vi "TMYTEK_FPGA_Ctrl.vi"() -> ()   [LabVIEW 2019]
uses:
  <vilib>/Platform/TimedLoop/XDataNode/timing_clust.ctl
  <vilib>/Platform/TimedLoop/XDataNode/nitl_modes.ctl
  <vilib>/Platform/TimedLoop/XDataNode/wakeup.ctl
  <vilib>/rvi/Emulation/niFpgaGetClockAttributes.vi
  <vilib>/rvi/Emulation/niFpgaSctlEmulationGetInTimedLoop.vi
  <vilib>/rvi/Emulation/niFpgaEmulationReportErrorSimple.vi
  <vilib>/rvi/eio/common/nirviEmuTemplateMethod_errors.vi
  <vilib>/rvi/Emulation/niFpgaCriticalErrorInLSC.vi
  <vilib>/rvi/interface/RandomDataEmulation/niFpgaRandomDataHandleErrors.vi
  <vilib>/eio/EIONode/EIONode.xnode
  <vilib>/platform/TimedLoop/XDataNode/XDataNode.xnode
  <vilib>/rvi/DataTransferAndStorage/Container/XNode/niFpgaContainer.xnode
  <vilib>/rvi/interface/RandomDataEmulation/nirviRandomDataFpgaReadWriteTemplate.vi
  <vilib>/Platform/TimedLoop/XDataNode/XDNodeRunTimeDep.lvlib
panel:
  in  "AUX I/O 7":bool
  in  "AUX I/O 6":bool
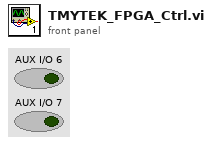
[diagram p1: front panel]
types:
  T1 = typedef "XDNodeRunTimeDep.lvlib/timing_clust.ctl" = cluster{"Expected End [f-1]":u64, "Actual End [f-1]":u64, "Finished Late? [f-1]":bool, "Expected End [i-1]":u64, "Actual End [i-1]":u64, "Finished Late? [i-1]":bool, "Expected Start [i]":u64, "Actual Start [i]":u64, "Expected Start [f]":u64, "Actual Start [f]":u64, "Source Name":string, "Structure Name":string, "Period":i64, "Deadline":i64, "Offset":i64, "Start":i64, "Priority":i32, "Timeout":i32, "Mode":T2, "Wakeup Reason":T3, "Error":errorcluster, "Source Type":string, "Secondary Source Type":string, "Global End Time":u64, "Global Start Time":u64, "Frame Duration":u64, "Iteration Duration":u64, "Assigned CPU":i32, "I/O Scan Engine Mode":u32}
  T2 = typedef "XDNodeRunTimeDep.lvlib/nitl_modes.ctl" = enum32{"No Change", "Process missed periods, maintain original phase", "Discard missed periods, maintain original phase", "Process missed periods, ignore original phase", "Discard missed periods, ignore original phase"}
  T3 = typedef "XDNodeRunTimeDep.lvlib/wakeup.ctl" = enum32{"Normal", "Aborted", "Asynchronous wakeup", "Timing source error", "Timed loop error", "Timeout"}
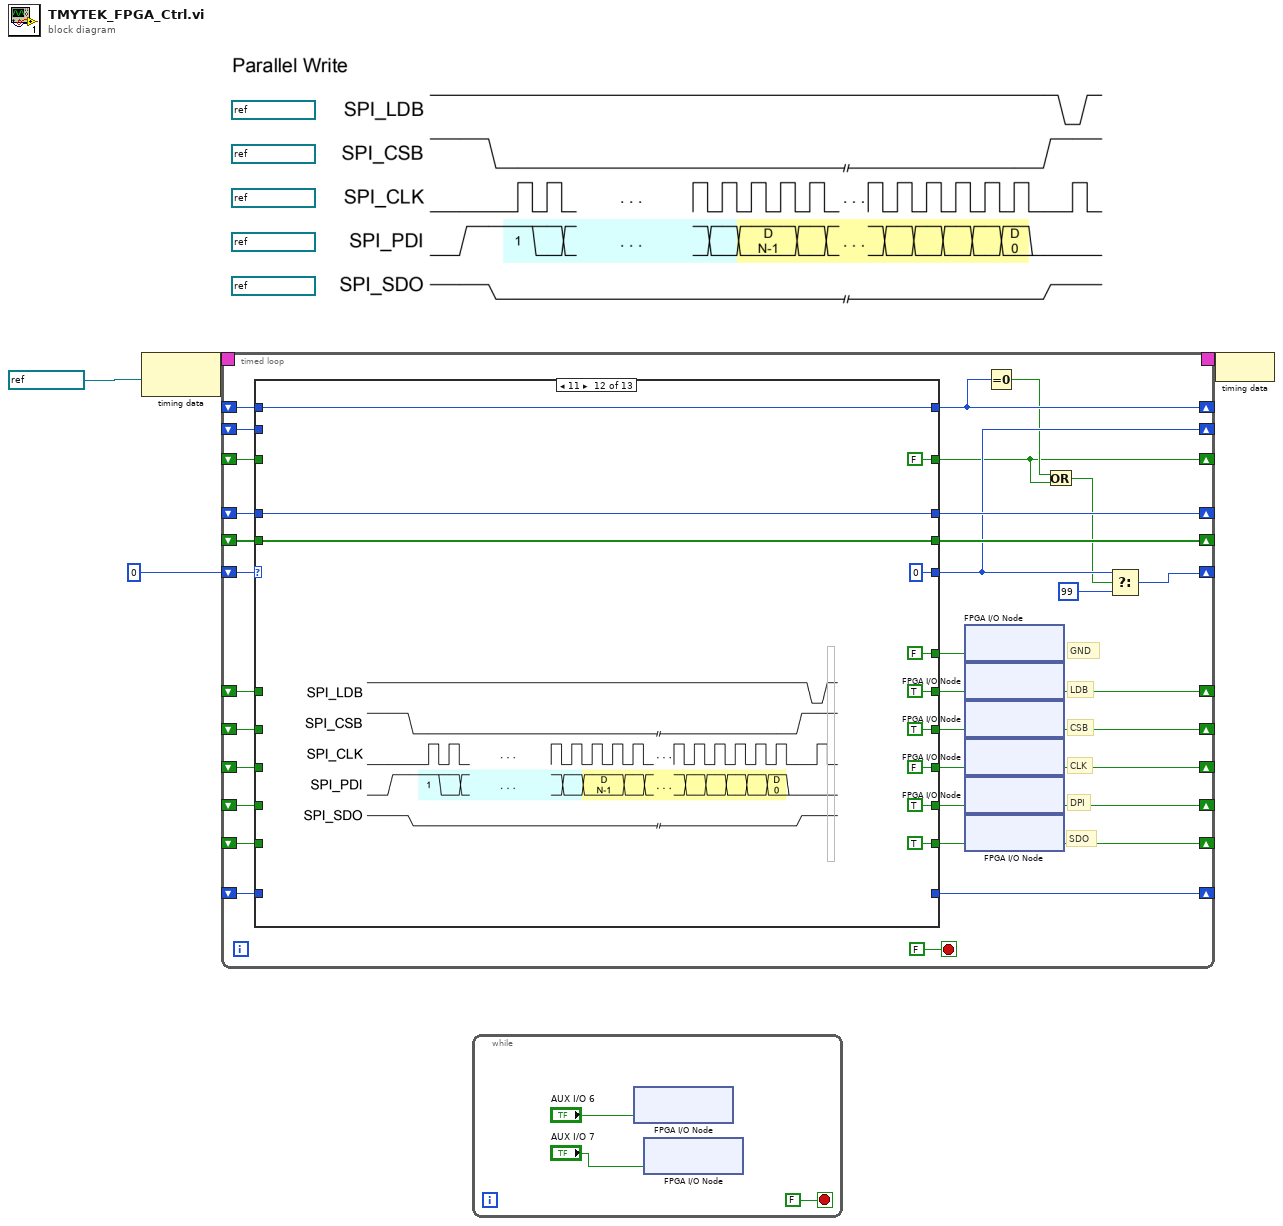
[diagram p0: block diagram]
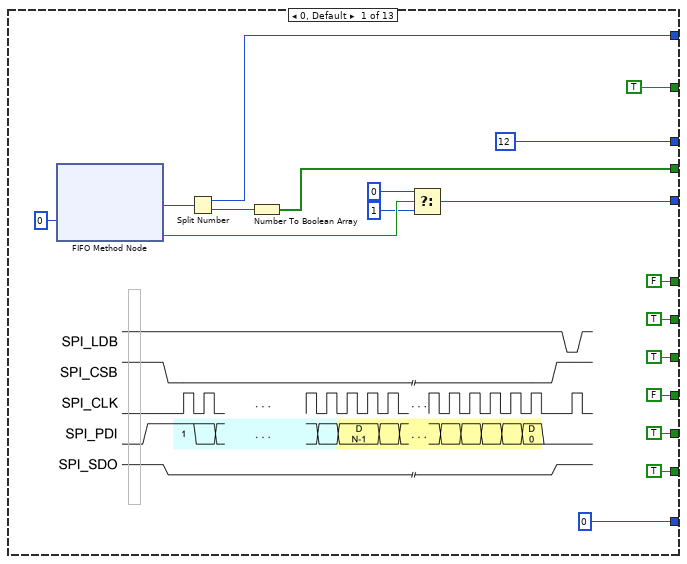
[diagram p2: hidden frame]
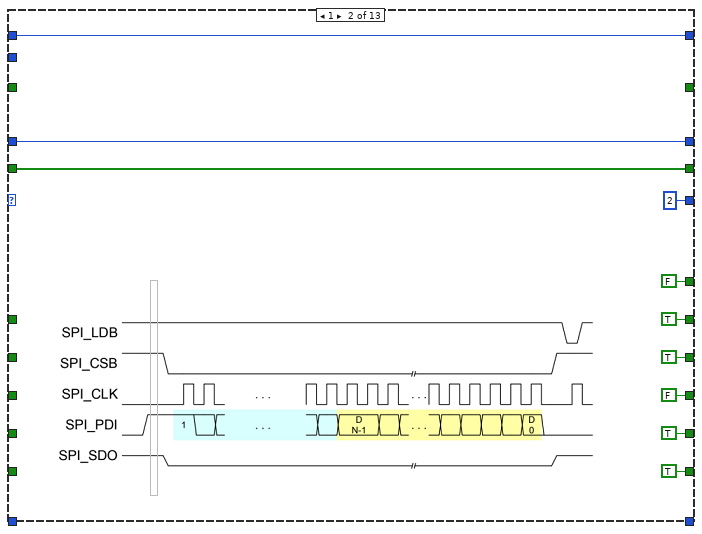
[diagram p3: hidden frame]
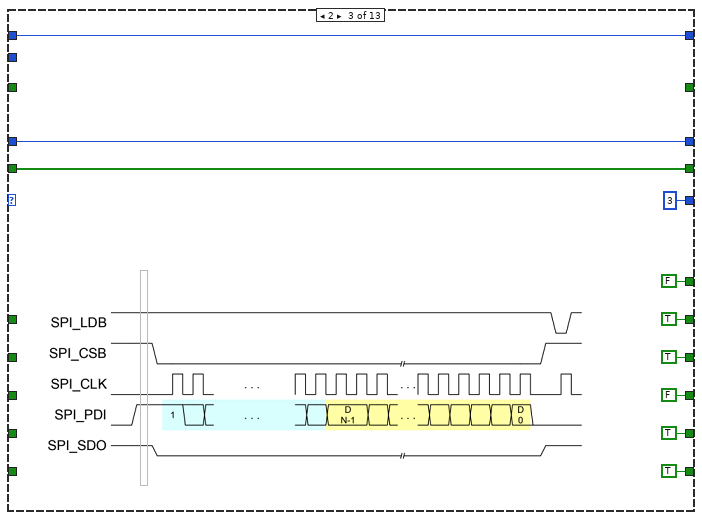
[diagram p4: hidden frame]
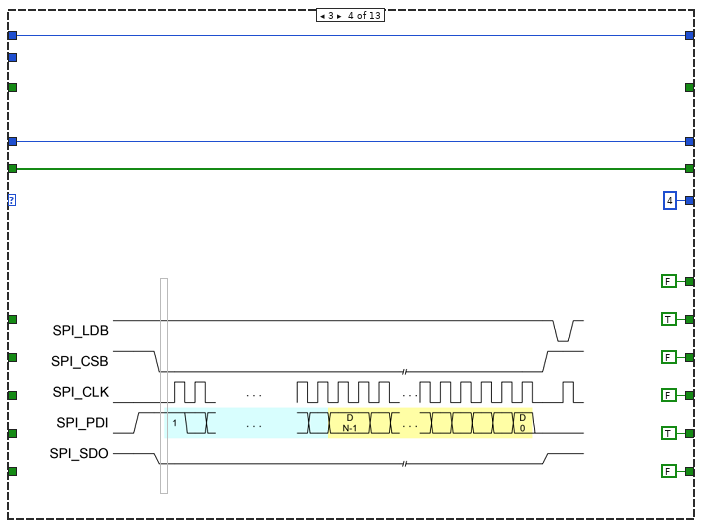
[diagram p5: hidden frame]
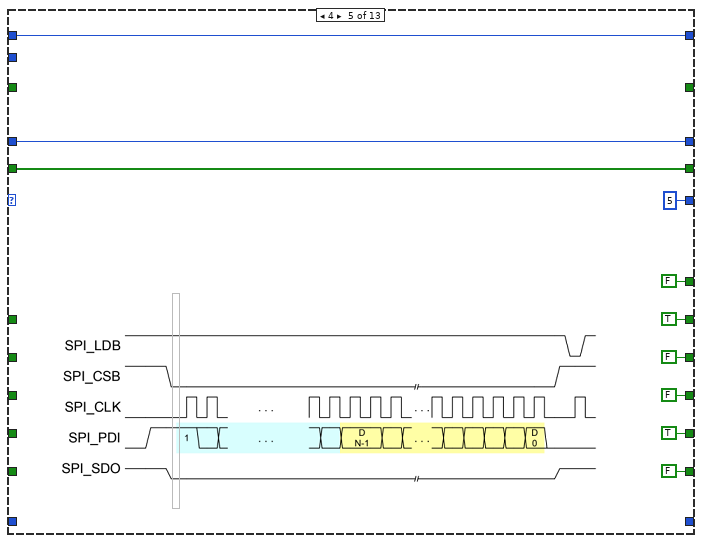
[diagram p6: hidden frame]
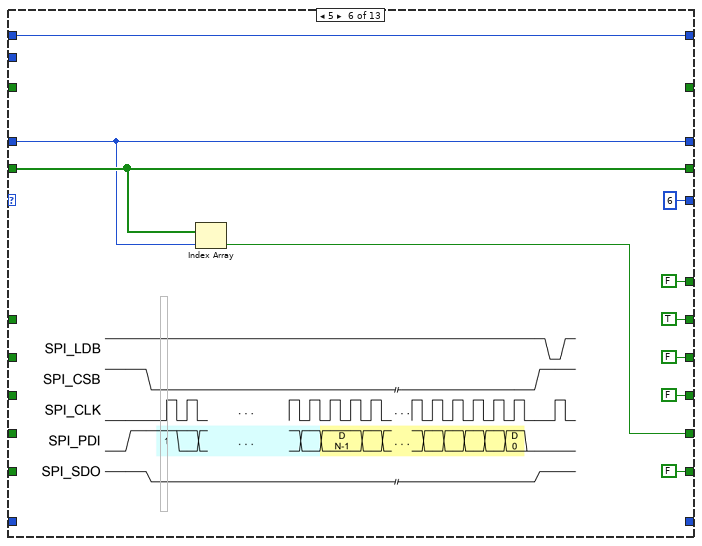
[diagram p7: hidden frame]
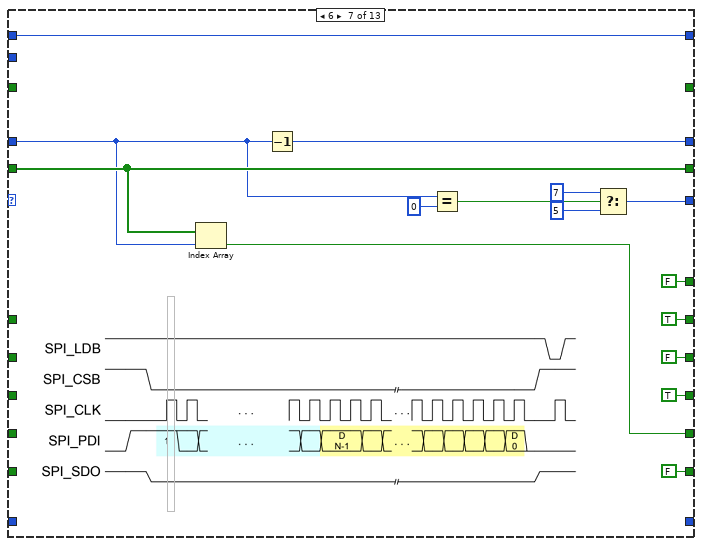
[diagram p8: hidden frame]
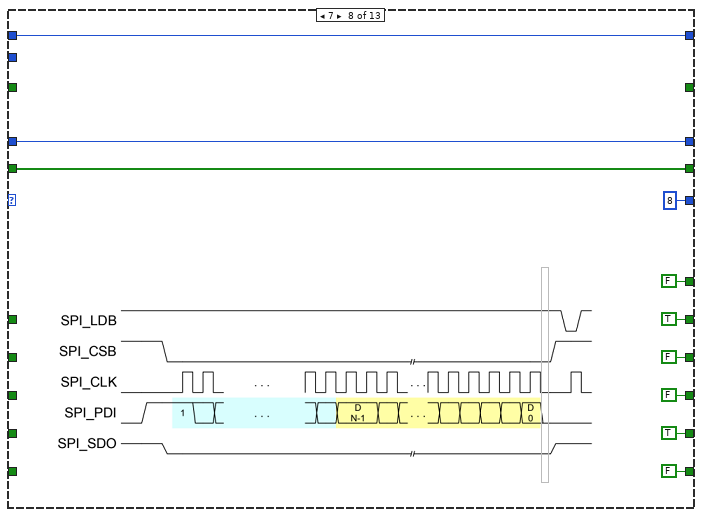
[diagram p9: hidden frame]
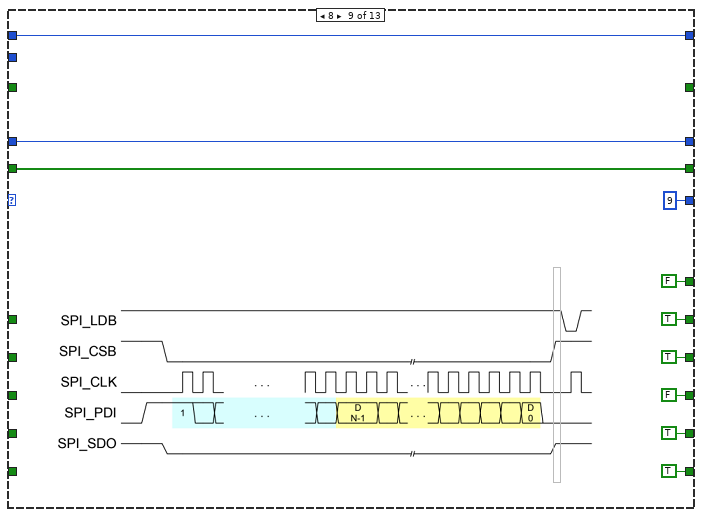
[diagram p10: hidden frame]
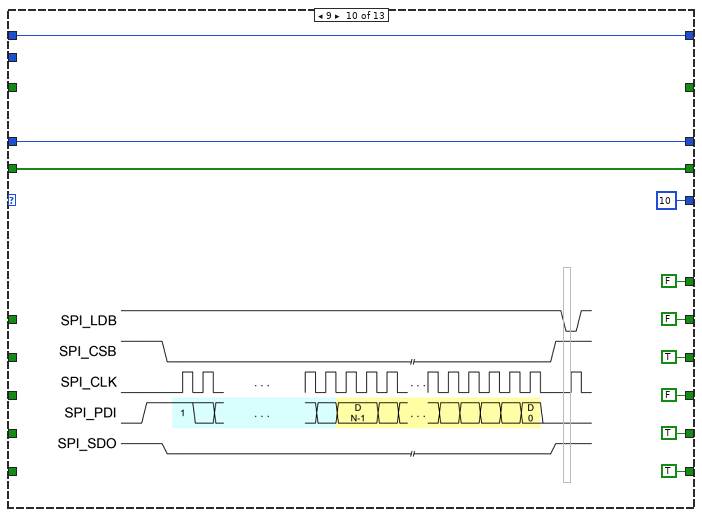
[diagram p11: hidden frame]
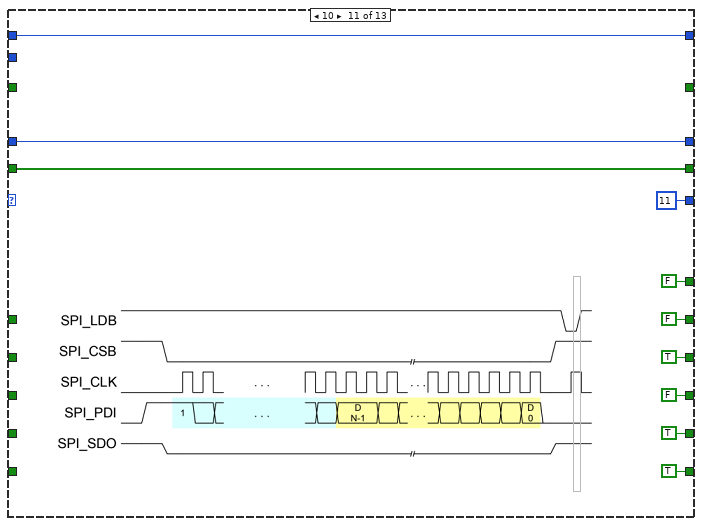
[diagram p12: hidden frame]
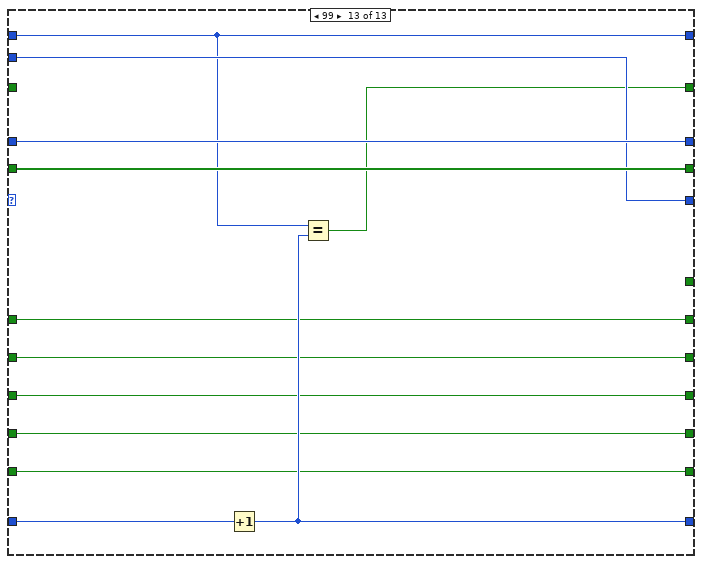
[diagram p13: hidden frame]
diagram:
  (unwired) refnum<k21> "AUX I/O 5" ("FPGA I/O")
  (unwired) refnum<k21> "AUX I/O 4" ("FPGA I/O")
  (unwired) refnum<k21> "AUX I/O 3" ("FPGA I/O")
  (unwired) refnum<k21> "AUX I/O 2" ("FPGA I/O")
  (unwired) refnum<k21> "AUX I/O 1" ("FPGA I/O")
  n1 = node-c288(refnum<k21> "120MHz" ("Source Name")) -> (w4:T1)
  n2 = timed-loop {
    timing: w4 -> [_]
    timing-out: [_] -> w3
    shift-right: [w24] -> _
    shift-left: i16 0 -> [w32]
    shift-right: [w31] -> _
    shift-left: _ -> [w30]
    shift-right: [w28] -> _
    shift-left: _ -> [w27]
    shift-right: [w23] -> _
    shift-left: _ -> [w22]
    shift-right: [w6] -> _
    shift-left: _ -> [w26]
    shift-right: [w21] -> _
    shift-left: _ -> [w20]
    shift-right: [w15] -> _
    shift-left: _ -> [w14]
    shift-right: [w16] -> _
    shift-left: _ -> [w13]
    shift-right: [w17] -> _
    shift-left: _ -> [w12]
    shift-right: [w18] -> _
    shift-left: _ -> [w11]
    shift-right: [w19] -> _
    shift-left: _ -> [w10]
    shift-right: [w8] -> _
    shift-left: _ -> [w9]
    stop <- FALSE stop-if-true
    # "SDO"
    # "DPI"
    # "CLK"
    # "GND"
    # "CSB"
    # "LDB"
    n3 = case shown="11" w32 {
      tunnel: [w47 i16 2 i16 3 i16 4 i16 5 i16 6 w103 i16 8 i16 9 i16 10 i16 11 i16 0 w177] -> w23
      tunnel: [w46 w61 w71 w81 w91 w99 w115 w119 w129 w139 w149 w160 w178] -> w31
      tunnel: w30 -> [_ w61 w71 w81 w91 w99 w115 w119 w129 w139 w149 w160 w178]
      tunnel: [FALSE FALSE FALSE FALSE FALSE FALSE FALSE FALSE FALSE FALSE FALSE FALSE _] -> w29
      tunnel: [TRUE TRUE TRUE TRUE TRUE TRUE TRUE TRUE TRUE FALSE FALSE TRUE w173] -> w15
      tunnel: [TRUE TRUE TRUE FALSE FALSE FALSE FALSE FALSE TRUE TRUE TRUE TRUE w172] -> w16
      tunnel: [FALSE FALSE FALSE FALSE FALSE FALSE TRUE FALSE FALSE FALSE FALSE FALSE w171] -> w17
      tunnel: [TRUE TRUE TRUE TRUE TRUE w97 w114 TRUE TRUE TRUE TRUE TRUE w170] -> w18
      tunnel: [TRUE TRUE TRUE FALSE FALSE FALSE FALSE FALSE TRUE TRUE TRUE TRUE w169] -> w19
      tunnel: [12 w55 w65 w77 w87 w98 w109 w126 w136 w146 w156 w167 w179] -> w28
      tunnel: w27 -> [_ w55 w65 w77 w87 w98 w108 w126 w136 w146 w156 w167 w179]
      tunnel: w26 -> [_ _ _ _ _ _ _ _ _ _ _ _ _]
      tunnel: [TRUE _ _ _ _ _ _ _ _ _ _ FALSE w174] -> w6
      tunnel: w22 -> [_ _ _ _ _ _ _ _ _ _ _ _ w177]
      tunnel: [u16 0 _ _ _ _ _ _ _ _ _ _ _ w175] -> w21
      tunnel: w20 -> [_ _ _ _ _ _ _ _ _ _ _ _ w176]
      tunnel: w14 -> [_ _ _ _ _ _ _ _ _ _ _ _ w173]
      tunnel: w13 -> [_ _ _ _ _ _ _ _ _ _ _ _ w172]
      tunnel: w12 -> [_ _ _ _ _ _ _ _ _ _ _ _ w171]
      tunnel: w11 -> [_ _ _ _ _ _ _ _ _ _ _ _ w170]
      tunnel: w10 -> [_ _ _ _ _ _ _ _ _ _ _ _ w169]
      tunnel: [w34 w52 w62 w72 w82 w92 w102 w117 w127 w137 w147 w158 w168] -> w8
      tunnel: w9 -> [_ w52 w62 w72 w82 w92 w102 w117 w127 w137 w147 w158 w168]
      frame 0, Default {
        n4 = xnode ("FIFO Method Node")("Timeout"=0) -> ("Element"=w36:u32, "Timed Out?"=w50:bool)  [unwired: 1 in, 1 out]
        n5 = Split Number(x=w36) -> (hi(x)=w34:u16, lo(x)=w35:u16)
        n6 = Number To Boolean Array(number=w35) -> (Boolean array=w46:bool[])
        n7 = Select(t=i16 0, s=w50, f=i16 1) -> (s? t:f=w47:i16)
      }
      frame 1 {
      }
      frame 2 {
      }
      frame 3 {
      }
      frame 4 {
      }
      frame 5 {
        n8 = Index Array(array=w99, index=w98) -> (element=w97:bool)
      }
      frame 6 {
        n9 = Index Array(array=w115, index=w108) -> (element=w114:bool)
        n10 = Decrement(x=w108) -> (x-1=w109:i32)
        n11 = Equal?(x=w108, y=0) -> (x = y?=w106:bool)
        n12 = Select(t=i16 7, s=w106, f=i16 5) -> (s? t:f=w103:i16)
      }
      frame 7 {
      }
      frame 8 {
      }
      frame 9 {
      }
      frame 10 {
      }
      frame 11 {
      }
      frame 99 {
        n13 = Increment(x=w176) -> (x+1=w175:u16)
        n14 = Equal?(x=w168, y=w175) -> (x = y?=w174:bool)
      }
    }
    n15 = xnode "FPGA I/O Node"("AUX I/O 0"=w29) -> ()  [unwired: 1 in, 1 out]
    n16 = xnode "FPGA I/O Node"("AUX I/O 1"=w15) -> ()  [unwired: 1 in, 1 out]
    n17 = xnode "FPGA I/O Node"("AUX I/O 2"=w16) -> ()  [unwired: 1 in, 1 out]
    n18 = xnode "FPGA I/O Node"("AUX I/O 3"=w17) -> ()  [unwired: 1 in, 1 out]
    n19 = xnode "FPGA I/O Node"("AUX I/O 4"=w18) -> ()  [unwired: 1 in, 1 out]
    n20 = xnode "FPGA I/O Node"("AUX I/O 5"=w19) -> ()  [unwired: 1 in, 1 out]
    n21 = Equal To 0?(x=w8) -> (x = 0?=w7:bool)
    n22 = Or(x=w7, y=w6) -> (x .or. y?=w5:bool)
    n23 = Select(t=w23, s=w5, f=i16 99) -> (s? t:f=w24:i16)
  }
  n24 = while {
    stop <- FALSE stop-if-true
    n25 = xnode "FPGA I/O Node"("AUX I/O 6"="AUX I/O 6") -> ()  [unwired: 1 in, 1 out]
    n26 = xnode "FPGA I/O Node"("AUX I/O 7"="AUX I/O 7") -> ()  [unwired: 1 in, 1 out]
  }
  n27 = node-c288(w3) -> ()
